vi "Bubble Sort Person Array Using Parameters.vi"(6 "Starting Month":u16(ring) items=["January", "February", "March", "April", "May", "June", "July", "August", "September", "October", "November", "December"], 8 "Reverse?":bool, 9 "Element Index":u8, 10 "Sort By":string="Default Order", 11 "Unsorted":T1[](array[typedef]) {"Birth Date" format="%<%Y/%b/%d>T"}) -> (3 "Sorted":T1[](array[typedef]) {"Birth Date" format="%<%Y/%b/%d>T"})   [LabVIEW 2023]
doc: "This VI implements a basic Bubble Sort for the array data, using the given parameters to decide how to do the sort. The \"Sort By\" string specifies how to sort. Depending upon the value of the string, different parameters are used:\n* \"Starting Month\" is used only if the \"Sort By\" string is \"Upcoming Birthday\". It specifies which month to start with for the sort. \n* \"Element Index\" is used only if the \"Sort By\" string is \"Nth Element\". It specifies which element of the cluster (cluster tab order) to use as the sort key."
uses:
  Person Information.ctl
panel:
  # "Look at all of these parameters. This connector pane is filling up fast!"
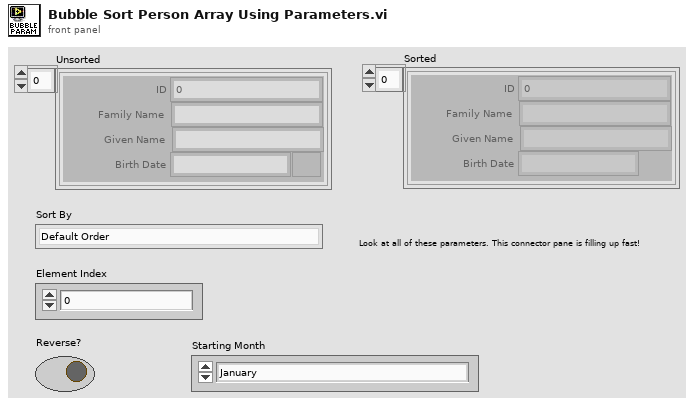
[diagram p1: front panel]
types:
  T1 = typedef "Person Information.ctl" = cluster{"ID":u32, "Family Name":string, "Given Name":string, "Birth Date":timestamp}
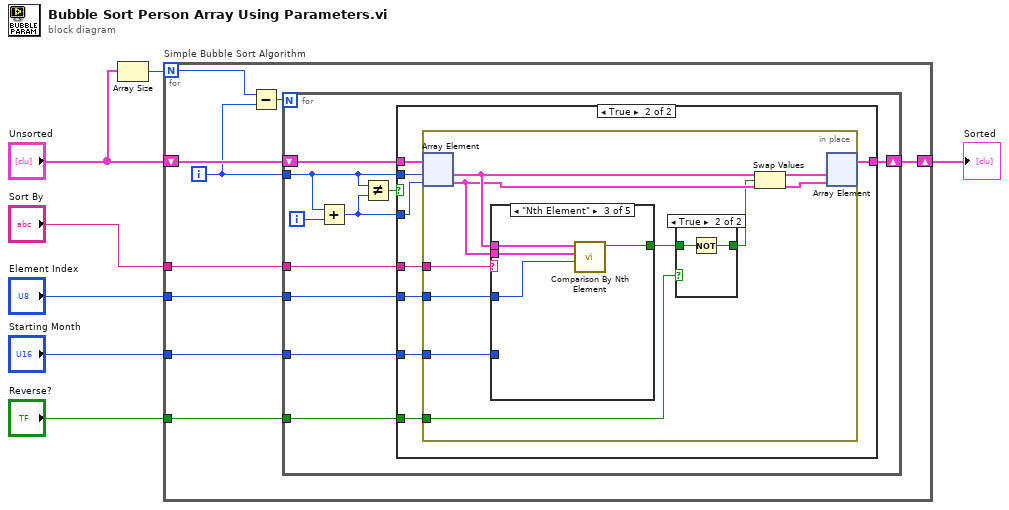
[diagram p0: block diagram]
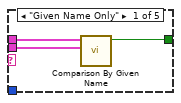
[diagram p4: hidden frame]
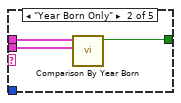
[diagram p5: hidden frame]
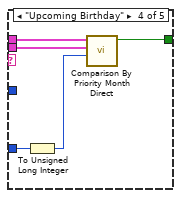
[diagram p6: hidden frame]
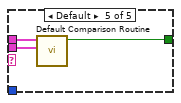
[diagram p7: hidden frame]
diagram:
  n1 = Array Size(array="Unsorted") -> (size(s)=w7:i32)
  n2 = for "Simple Bubble Sort Algorithm" {
    N: w7 -> [w13]
    shift-right: [w15] -> w6
    shift-left: "Unsorted" -> [w16]
    tunnel: "Sort By" -> [w11]
    tunnel: "Reverse?" -> [w10]
    tunnel: "Element Index" -> [w9]
    tunnel: "Starting Month" -> [w8]
    i -> [w12]
    n3 = Subtract(x=w13, y=w12) -> (x-y=w14:i32)
    n4 = for {
      N: w14 -> [_]
      shift-right: [w25] -> w15
      shift-left: w16 -> [w26]
      tunnel: w12 -> [w21]
      tunnel: w11 -> [w20]
      tunnel: w10 -> [w19]
      tunnel: w9 -> [w18]
      tunnel: w8 -> [w17]
      i -> [w23]
      n5 = Add(x=w21, y=w23) -> (x+y=w22:i32)
      n6 = Not Equal?(x=w21, y=w22) -> (x != y?=w24:bool)
      n7 = case shown="True" w24 {
        tunnel: w26 -> [w27 w35]
        tunnel: [w27 w34] -> w25
        tunnel: w21 -> [_ w33]
        tunnel: w22 -> [_ w32]
        tunnel: w20 -> [_ w31]
        tunnel: w19 -> [_ w30]
        tunnel: w18 -> [_ w29]
        tunnel: w17 -> [_ w28]
        frame False {
        }
        frame True {
          n8 = in-place {
            in-place-border: w31 -> [w41]
            in-place-border: w30 -> [w38]
            in-place-border: w29 -> [w37]
            in-place-border: w28 -> [w36]
            n9 = in-place-array #1(w35, w33, w32) -> (w43:T1, w42:T1)
            n10 = case shown="\"Nth Element\"" w41 {
              tunnel: w43 -> [w51 w54 w58 w63 w66]
              tunnel: w42 -> [w50 w52 w57 w62 w65]
              tunnel: [w49 w53 w56 w61 w64] -> w39
              tunnel: w37 -> [_ _ w55 _ _]
              tunnel: w36 -> [_ _ _ w60 _]
              frame "Given Name Only" {
                n11 = call "Comparison By Given Name.vi"("Person B"=w50, "Person A"=w51) -> ("Swap?"=w49:bool)  [unwired: 9 in]
              }
              frame "Year Born Only" {
                n12 = call "Comparison By Year Born.vi"("Person B"=w52, "Person A"=w54) -> ("Swap?"=w53:bool)  [unwired: 9 in]
              }
              frame "Nth Element" {
                n13 = call "Comparison By Nth Element.vi"("Element Index"=w55, "Person B"=w57, "Person A"=w58) -> ("Swap?"=w56:bool)  [unwired: 8 in]
              }
              frame "Upcoming Birthday" {
                n14 = To Unsigned Long Integer(number=w60) -> (unsigned 32bit integer=w59:u32)
                n15 = call "Comparison By Priority Month Direct.vi"("Starting Month"=w59, "Person B"=w62, "Person A"=w63) -> ("Swap?"=w61:bool)  [unwired: 8 in]
              }
              frame Default {
                n16 = call "Default Comparison Routine.vi"("Person B"=w65, "Person A"=w66) -> ("Swap?"=w64:bool)  [unwired: 9 in]
              }
            }
            n17 = case shown="True" w38 {
              tunnel: [w46 w48] -> w40
              tunnel: w39 -> [w46 w47]
              frame False {
              }
              frame True {
                n18 = Not(x=w47) -> (.not. x?=w48:bool)
              }
            }
            n19 = Swap Values(12:w43, 13:w40, 14:w42) -> (1:w45:T1, 3:w44:T1)
            n20 = in-place-array #1(w45, w44) -> (w34:T1[])  [unwired: 2 out]
          }
        }
      }
    }
  }
  "Sorted" <- w6
